vi "Update GUI Element.vi"(8 "error in (no error)":errorcluster, 11 "Sequencing Control in":refnum<class "Sequencing Control.lvclass">) -> (0 "error out":errorcluster, 3 "Sequencing Control out":refnum<class "Sequencing Control.lvclass">)   [LabVIEW 2023, in "VolatusSeqGUI.lvlib" / "Sequencing Control.lvclass"]
uses:
  Sequencing Control.lvclass
  VolatusGUI/GUI Element/GUI Element.lvclass/GUI Element.ctl
  Sequencing Control.lvclass/Sequencing Control.ctl
  lv-vecto/Vecto/Unix ns to Double Timestamp.vi
  lv-vecto/Vecto/Relative ns to Double Seconds.vi
  VolatusGUIElements/VolatusGUIElements.lvlib
  VolatusGUI/GUI Element/GUI Element.lvclass
  C:/dev/volatus/mts-volatus-super/libs/lv-volatus/VolatusGUI/GUI Element/GUI Element.lvclass
  C:/dev/volatus/mts-volatus-super/libs/lv-volatus/VolatusSeqGUI/Sequencing Control/Sequencing Control.lvclass
  C:/dev/volatus/mts-volatus-super/libs/lv-volatus/VolatusGUI/OnValueChangeHandler/OnValueChangeHandler.lvclass
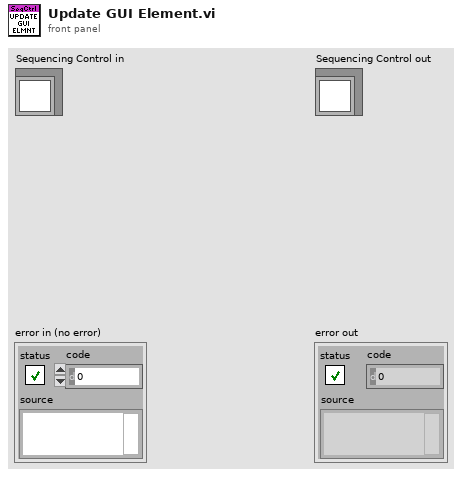
[diagram p1: front panel]
types:
  T1 = cluster{"Sequences":cluster{"Name Color":u32, "Name":string, "Btn 1 Color":u32, "Btn 1 Text":string, "Btn 2 Color":u32, "Btn 2 Text":string, "Status Color":u32, "Status":string, "State Time":string, "Started":string, "Seq Time":string, "Btn 1":bool, "Btn 2":bool, "Btn Name":bool}[], "Unload All":bool, "Abort All":bool, "Loaded, Good CRC":u32, "Sequence Error":u32, "Loaded, CRC Mismatch":u32, "Running, Good CRC":u32, "Unloaded":u32, "Running, CRC Mismatch":u32}
  T2 = typedef "VolatusSeq.lvlib/Sequence Status JSON.ctl" = cluster{"name":string, "state":string, "running":bool, "abort":bool, "time":cluster{"seq":i64, "state":i64, "wall":i64}, "loaded":bool, "started":i64, "crc":u32, "color_bg":string, "error":errorcluster, "period":i64, "late":bool}
  T3 = typedef "VolatusSeqGUI.lvlib/Sequencing Control.lvclass/Local File Info.ctl" = cluster{"Path":path, "Name":string, "CRC":u32, "Last Modified":timestamp, "error":errorcluster}
  T4 = typedef "VolatusSeqGUI.lvlib/Sequencing Control.lvclass/Colors.ctl" = cluster{"Default":u32, "Unloaded":u32, "Seq Error":u32, "Loaded Good CRC":u32, "Loaded Bad CRC":u32, "Running Good CRC":u32, "Running Bad CRC":u32}
  T5 = cluster{"Name":string, "Status":T2, "CRC":u32, "status":bool, "Exists Locally":bool}
  T6 = cluster{"name":string, "Status":T2, "Info.CRC":u32, bool, "Exists Locally":bool}
  T7 = cluster{"Name":string, "Status":T2, "CRC":u32, "status":bool, "Exists Locally":bool}[]
  T8 = cluster{"Name Color":u32, "Name":string, "Btn 1 Color":u32, "Btn 1 Text":string, "Btn 2 Color":u32, "Btn 2 Text":string, "Status Color":u32, "Status":string, "State Time":string, "Started":string, "Seq Time":string, "Btn 1":bool, "Btn 2":bool, "Btn Name":bool}
  T9 = typedef "VolatusSeqGUI.lvlib/Sequencing Control.lvclass/Sequence Status.ctl" = enum16{"Unloaded Not Local", "Unloaded", "Load Error", "Loaded Good CRC", "Loaded Bad CRC", "Running Good CRC", "Running Bad CRC", "Local Error"}
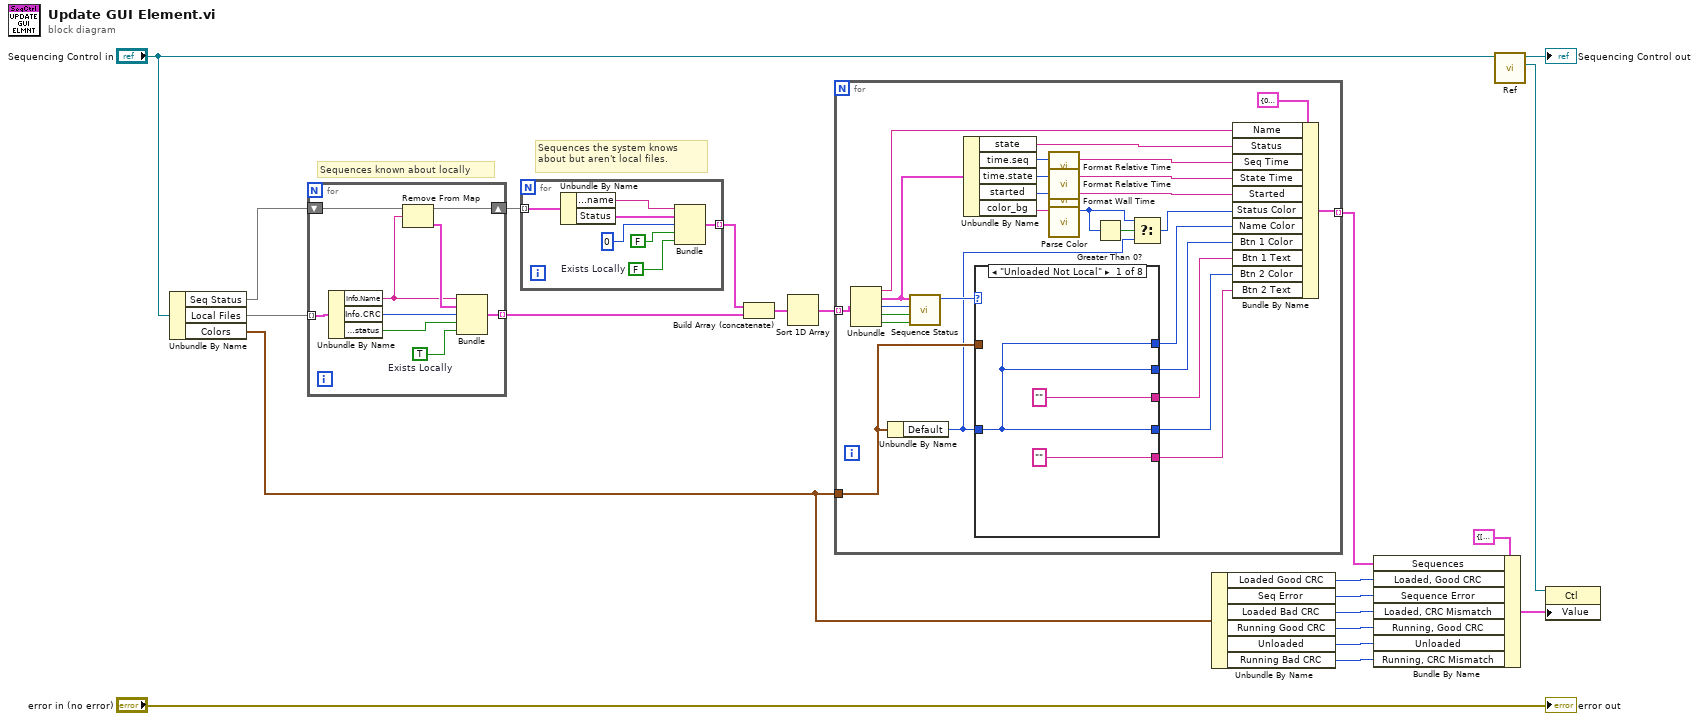
[diagram p0: block diagram]
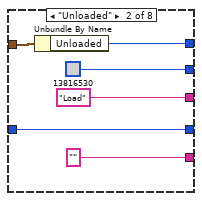
[diagram p2: hidden frame]
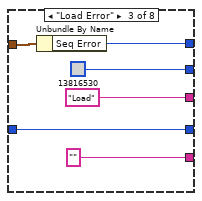
[diagram p3: hidden frame]
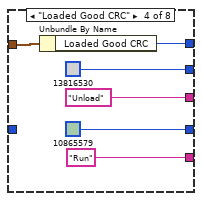
[diagram p4: hidden frame]
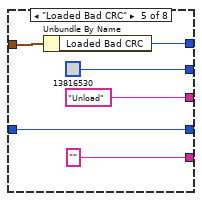
[diagram p5: hidden frame]
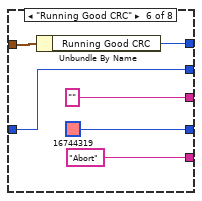
[diagram p6: hidden frame]
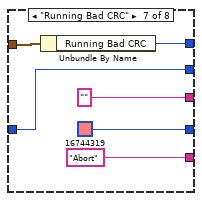
[diagram p7: hidden frame]
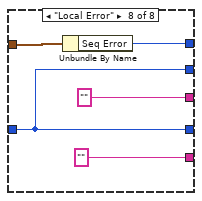
[diagram p8: hidden frame]
diagram:
  # "Sequences the system knows about but aren't local files."
  # "Sequences known about locally"
  n1 = Unbundle By Name("Sequencing Control in") -> ("Seq Status"=w14:map{string, T2}, "Local Files"=w1:map{path, T3}, "Colors"=w11:T4)
  n2 = for {
    tunnel: w1 -> [w30] mode=indexing
    shift-right: [w28] -> w19
    shift-left: w14 -> [w29]
    tunnel: [w25] -> w17 mode=indexing
    w22 = TRUE  # Exists Locally
    n3 = Unbundle By Name(w30) -> ("Info.Name"=w23:string, "Info.CRC"=w27:u32, "Info.error.status"=w24:bool)
    n4 = Remove From Map(10:w23, 11:w29) -> (1:w26:T2, 3:w28:map{string, T2})  [unwired: 1 out]
    n5 = Bundle("Name"=w23, "Status"=w26, "CRC"=w27, "status"=w24, "Exists Locally"=w22) -> (w25:T5)  [unwired: 1 in]
  }
  n6 = for {
    tunnel: w19 -> [w36] mode=indexing
    tunnel: [w34] -> w18 mode=indexing
    w31 = FALSE  # Exists Locally
    n7 = Unbundle By Name(w36) -> ("Status.name"=w37:string, "Status"=w33:T2)
    n8 = Bundle("name"=w37, "Status"=w33, "Info.CRC"=u32 0, FALSE, "Exists Locally"=w31) -> (w34:T6)  [unwired: 1 in]
  }
  n9 = Build Array (concatenate)(w18, w17) -> (w16:T7)
  n10 = Sort 1D Array(array=w16) -> (sorted array=w15:T7)
  n11 = for {
    tunnel: w15 -> [w64] mode=indexing
    tunnel: w11 -> [w45]
    tunnel: [w51] -> w12 mode=indexing
    n12 = Unbundle(w64) -> ("Name"=w46:string, "Status"=w39:T2, "CRC"=w63:u32, "status"=w40:bool, "Exists Locally"=w38:bool)
    n13 = Unbundle By Name(w45) -> ("Default"=w42:u32)
    n14 = call "Sequence Status.vi"("Exists Locally"=w38, "Local Error"=w40, "Local CRC"=w63, "Sequence Status JSON"=w39) -> ("Sequence Status"=w61:T9)  [unwired: 7 in]
    n15 = Unbundle By Name(w39) -> ("state"=w58:string, "time.seq"=w56:i64, "time.state"=w57:i64, "started"=w53:i64, "color_bg"=w59:string)
    n16 = case shown="\"Unloaded Not Local\"" w61 {
      tunnel: w45 -> [_ w73 w79 w85 w91 w97 w103 w108]
      tunnel: [w65 w72 w78 w84 w90 w96 w102 w107] -> w60
      tunnel: [w65 u32 13816530 u32 13816530 u32 13816530 u32 13816530 w92 w98 w104] -> w50
      tunnel: ["" "Load" "Load" "Unload" "Unload" "" "" ""] -> w49
      tunnel: [w65 w68 w75 u32 10865579 w86 u32 16744319 u32 16744319 w104] -> w48
      tunnel: ["" "" "" "Run" "" "Abort" "Abort" ""] -> w47
      tunnel: w42 -> [w65 w68 w75 _ w86 w92 w98 w104]
      frame "Unloaded Not Local" {
      }
      frame "Unloaded" {
        n17 = Unbundle By Name(w73) -> ("Unloaded"=w72:u32)
      }
      frame "Load Error" {
        n18 = Unbundle By Name(w79) -> ("Seq Error"=w78:u32)
      }
      frame "Loaded Good CRC" {
        n19 = Unbundle By Name(w85) -> ("Loaded Good CRC"=w84:u32)
      }
      frame "Loaded Bad CRC" {
        n20 = Unbundle By Name(w91) -> ("Loaded Bad CRC"=w90:u32)
      }
      frame "Running Good CRC" {
        n21 = Unbundle By Name(w97) -> ("Running Good CRC"=w96:u32)
      }
      frame "Running Bad CRC" {
        n22 = Unbundle By Name(w103) -> ("Running Bad CRC"=w102:u32)
      }
      frame "Local Error" {
        n23 = Unbundle By Name(w108) -> ("Seq Error"=w107:u32)
      }
    }
    n24 = call "Format Relative Time.vi"("Unix ns"=w56) -> ("String"=w55:string)  [unwired: 6 in]
    n25 = call "Format Relative Time.vi"("Unix ns"=w57) -> ("String"=w54:string)  [unwired: 6 in]
    n26 = call "Format Wall Time.vi"("Unix ns"=w53) -> ("String"=w52:string)  [unwired: 6 in]
    n27 = call "Parse Color.vi"("Color String"=w59) -> ("Color"=w43:u32)  [unwired: 9 in, 1 out]
    n28 = Greater Than 0?(x=w43) -> (x > 0?=w44:bool)
    n29 = Select(t=w43, s=w44, f=w42) -> (s? t:f=w41:u32)
    n30 = Bundle By Name(cluster=T8 {"Name Color"=0, "Name"="", "Btn 1 Color"=0, "Btn 1 Text"="", "Btn 2 Color"=0, "Btn 2 Text"="", "Status Color"=0, "Status"="", "State Time"="", "Started"="", "Seq Time"="", "Btn 1"=FALSE, "Btn 2"=FALSE, "Btn Name"=FALSE} ("Sequence"), "Name"=w46, "Status"=w58, "Seq Time"=w55, "State Time"=w54, "Started"=w52, "Status Color"=w41, "Name Color"=w60, "Btn 1 Color"=w50, "Btn 1 Text"=w49, "Btn 2 Color"=w48, "Btn 2 Text"=w47) -> (w51:T8)
  }
  n31 = Unbundle By Name(w11) -> ("Loaded Good CRC"=w10:u32, "Seq Error"=w9:u32, "Loaded Bad CRC"=w8:u32, "Running Good CRC"=w7:u32, "Unloaded"=w6:u32, "Running Bad CRC"=w5:u32)
  n32 = Bundle By Name(cluster=T1 {"Sequences"=[], "Unload All"=FALSE, "Abort All"=FALSE, "Loaded, Good CRC"=13816530, "Sequence Error"=16744319, "Loaded, CRC Mismatch"=16777142, "Running, Good CRC"=11730866, "Unloaded"=7171459, "Running, CRC Mismatch"=10530559} ("Sequencing"), "Sequences"=w12, "Loaded, Good CRC"=w10, "Sequence Error"=w9, "Loaded, CRC Mismatch"=w8, "Running, Good CRC"=w7, "Unloaded"=w6, "Running, CRC Mismatch"=w5) -> (w2:T1)
  n33 = call "Ref.vi"("GUI Element in"="Sequencing Control in") -> ("Ref"=w3:refnum<vi>, "GUI Element out"=→"Sequencing Control out":refnum<class "Sequencing Control.lvclass">)  [unwired: 9 in]
  n34 = property class="Ctl"(reference=w3, "Value"=w2) -> ()  [unwired: 1 in, 2 out]
  "error out" <- "error in (no error)"
